vi "水温校准.vi"() -> ()   [LabVIEW 2016, in "斯坦道多参数.lvlib"]
uses:
  <vilib>/Utility/miscctls.llb/LVPointTypeDef.ctl
  <vilib>/Utility/miscctls.llb/LVPositionTypeDef.ctl
  <vilib>/Utility/miscctls.llb/LVBoundsTypeDef.ctl
  <vilib>/Utility/config.llb/NI_LVConfig.lvlib
panel:
  out "字符串":string
  in  "补偿后温度值":dbl format="%#_g ℃"
  out "电极温度读值":dbl format="%#_g ℃"
  in  "温度偏移补偿":dbl format="%#_g ℃"
  in  "温度电极选择":enum16{"pH电极", "电导率电极", "溶解氧电极", "浊度电极"}(ring)
  # "温度电极设定"
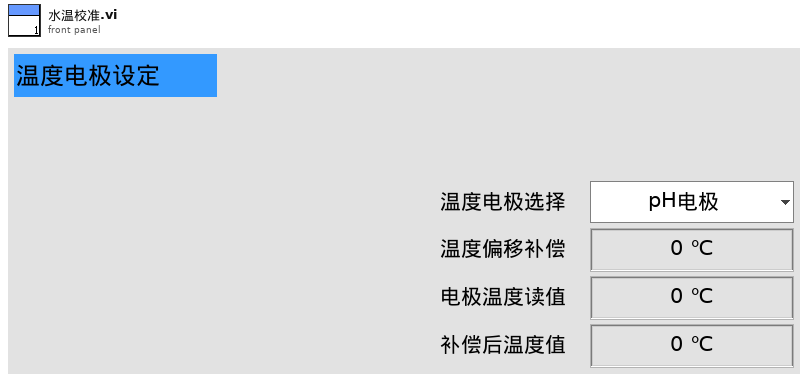
[diagram p1: front panel]
types:
  T1 = typedef "LVPointTypeDef.ctl" = cluster{"Horizontal":i16, "Vertical":i16}
  T2 = typedef "LVPositionTypeDef.ctl" = cluster{"Left":i32, "Top":i32}
  T3 = typedef "LVBoundsTypeDef.ctl" = cluster{"Width":u32, "Height":u32}
  T4 = cluster{"pH探头选择":u16, "DO探头选择":u16, "电导率探头选择":u16, "浊度探头选择":u16, "叶绿素a探头选择":u16, "蓝绿藻探头选择":u16, "orp探头选择":u16}
  T5 = cluster{"CH":u16, "监测值":dbl, "温度偏移修正值":sgl, "信号值":sgl}
  T6 = typedef "NI_LVConfig.lvlib/Config Data RefNum.ctl" = refnum<k1>
  T7 = cluster{"报警码":u16, "pH数值":sgl, "0X0003_NC":sgl, "温度数据":sgl, "pH原始信号 mv":sgl, "0X0009_NC":string, "产品名称":string, "序列号":string, "硬件版本":string, "软件版本":string, "通讯地址":u16, "波特率":u16, "设备类型":u16, "0X0026_NC":string, "第一点原始数据":sgl, "第一点校准数据":sgl, "第二点原始数据":sgl, "第二点校准数据":sgl, "探头校准命令":u16, "温度校准参数":sgl, "温度校准命令":u16}
  T8 = cluster{"报警码":u16, "电导率数据（uS/cm）":sgl, "0x0003 NC":sgl, "温度数据":sgl, "电导率原始信号电阻":sgl, "当前量程":u16, "温度补偿系数":sgl, "0X0009_NC":string, "产品名称":string, "序列号":string, "硬件版本":string, "软件版本":string, "通讯地址":u16, "波特率":u16, "设备类型":u16, "0X0026_NC":string, "第一点原始数据":sgl, "第一点校准数据":sgl, "0X0035_NC":sgl, "0X0037_NC":sgl, "探头校准命令":u16, "温度校准参数":sgl, "温度校准命令":u16}
  T9 = cluster{"报警码":u16, "溶解氧数值（mg/L）":sgl, "溶解氧数据（%）":sgl, "温度数据":sgl, "溶解氧原始信号 nA":sgl, "大气压力":sgl, "盐度":sgl, "0X0009_NC":string, "产品名称":string, "序列号":string, "硬件版本":string, "软件版本":string, "通讯地址":u16, "波特率":u16, "设备类型":u16, "0X0026_NC":string, "第一点原始数据":sgl, "第一点校准数据":sgl, "第二点原始数据":sgl, "第二点校准数据":sgl, "探头校准命令":u16, "温度校准参数":sgl, "温度校准命令":u16}
  T10 = cluster{"报警码":u16, "浊度数值 NTU":sgl, "温度数据":sgl, "原始光强数值":u16, "量程":u16, "平均次数":u16, "清扫模式":u16, "清扫次数":u16, "清扫间隔分钟":u16, "0X000B_NC":string, "产品名称":string, "序列号":string, "硬件版本":string, "软件版本":string, "通讯地址":u16, "波特率":u16, "设备类型":u16, "0X0026_NC":string, "校准量程":u16, "第一点原始光强":u16, "第一点校准数据":sgl, "第二点原始光强":u16, "第二点校准数据":sgl, "第三点原始光强":u16, "第三点校准数据":sgl, "探头校准命令":u16, "温度校准参数":sgl, "温度校准命令":u16}
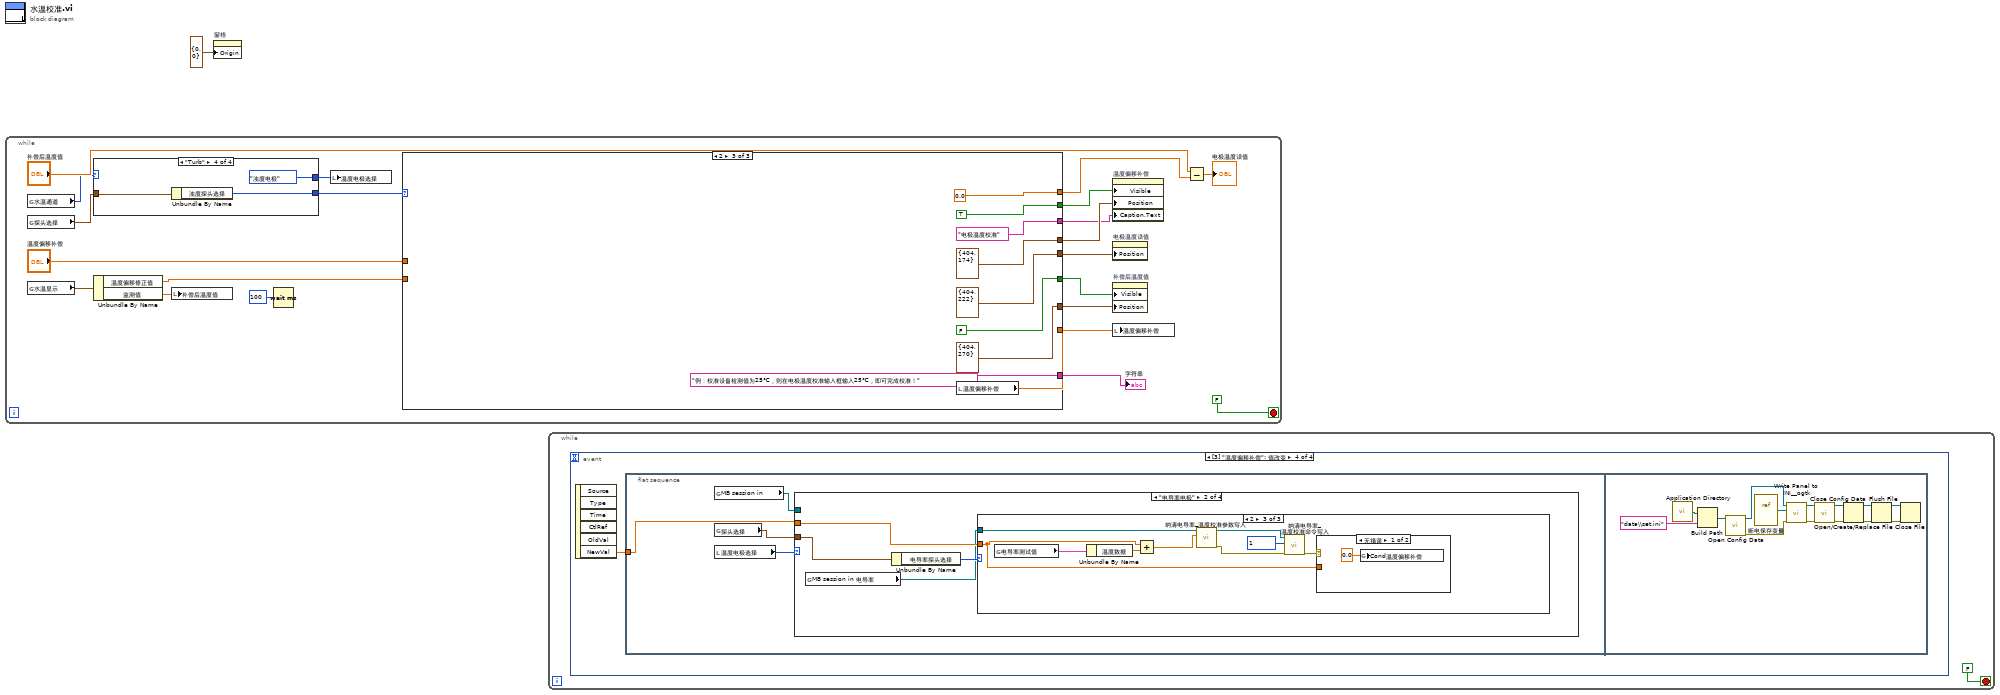
[diagram p0: block diagram]
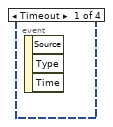
[diagram p2: hidden frame]
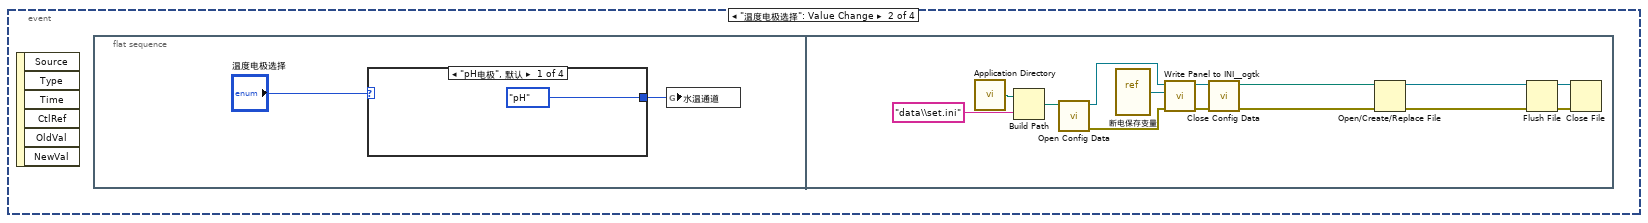
[diagram p3: hidden frame]
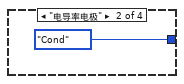
[diagram p4: hidden frame]
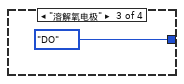
[diagram p5: hidden frame]
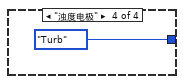
[diagram p6: hidden frame]
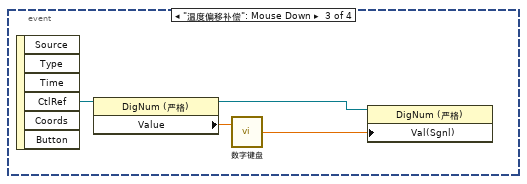
[diagram p7: hidden frame]
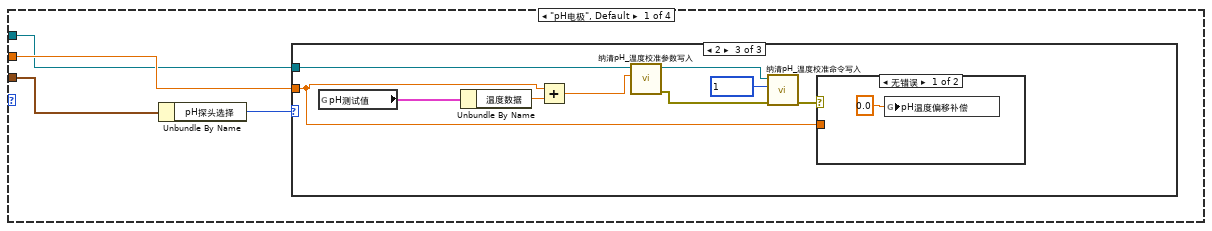
[diagram p8: hidden frame]
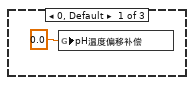
[diagram p9: hidden frame]
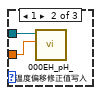
[diagram p10: hidden frame]
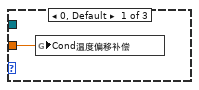
[diagram p12: hidden frame]
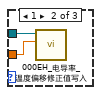
[diagram p13: hidden frame]
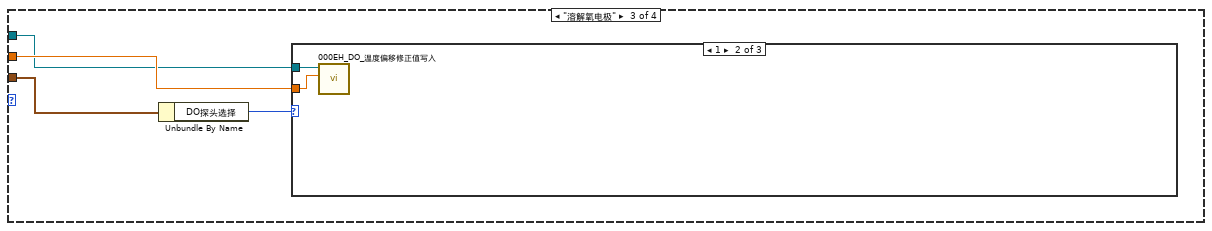
[diagram p15: hidden frame]
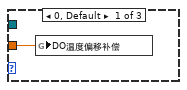
[diagram p16: hidden frame]
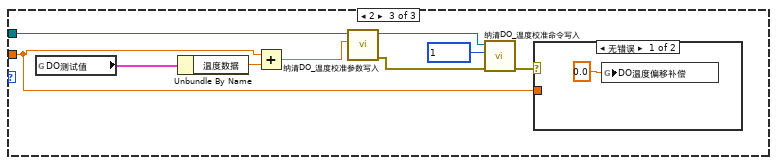
[diagram p17: hidden frame]
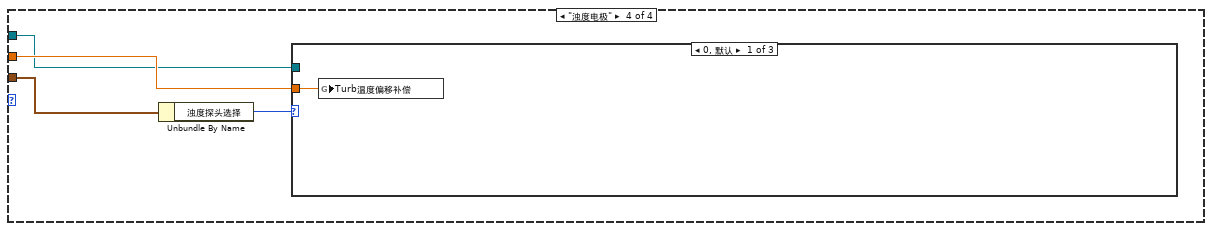
[diagram p19: hidden frame]
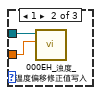
[diagram p20: hidden frame]
diagram:
  n1 = while {
    stop <- FALSE stop-if-true
    n2 = global read "断电保存变量.vi" "水温通道"() -> (w17:enum16{"pH", "Cond", "DO", "Turb"})
    n3 = global read "断电保存变量.vi" "探头选择"() -> (w14:T4)
    n4 = global read "多参数全局变量.vi" "水温显示"() -> (w16:T5)
    n5 = case shown="\"Turb\"" w17 {
      tunnel: [enum16{"pH电极", "电导率电极", "溶解氧电极", "浊度电极"}."pH电极" ("温度电极选择") enum16{"pH电极", "电导率电极", "溶解氧电极", "浊度电极"}."电导率电极" ("温度电极选择") enum16{"pH电极", "电导率电极", "溶解氧电极", "浊度电极"}."溶解氧电极" ("温度电极选择") enum16{"pH电极", "电导率电极", "溶解氧电极", "浊度电极"}."浊度电极" ("温度电极选择")] -> w15
      tunnel: w14 -> [w50 w53 w56 w59]
      tunnel: [w49 w52 w55 w58] -> w13
      frame "pH", Default {
        n6 = Unbundle By Name(w50) -> ("pH探头选择"=w49:u16)
      }
      frame "Cond" {
        n7 = Unbundle By Name(w53) -> ("电导率探头选择"=w52:u16)
      }
      frame "DO" {
        n8 = Unbundle By Name(w56) -> ("DO探头选择"=w55:u16)
      }
      frame "Turb" {
        n9 = Unbundle By Name(w59) -> ("浊度探头选择"=w58:u16)
      }
    }
    n10 = Unbundle By Name(w16) -> ("温度偏移修正值"=w6:sgl, "监测值"=w18:dbl)
    n11 = local write "补偿后温度值"(w18) -> ()
    n12 = Wait (ms)(milliseconds to wait=u32 100 ("等待时间（毫秒）")) -> ()  [unwired: 1 out]
    n13 = local write "温度电极选择"(w15) -> ()
    n14 = case shown="2" w13 {
      tunnel: [FALSE ("可见") TRUE ("可见") TRUE ("可见")] -> w12
      tunnel: [w29 T2 {"Left"=404, "Top"=174} ("位置") T2 {"Left"=404, "Top"=174} ("位置")] -> w11
      tunnel: [w29 T3 {"Width"=404, "Height"=222} ("边界") T3 {"Width"=404, "Height"=222} ("边界")] -> w10
      tunnel: [FALSE ("可见") TRUE ("可见") FALSE ("可见")] -> w9
      tunnel: [T2 {"Left"=404, "Top"=270} ("位置 2") T2 {"Left"=404, "Top"=270} ("位置 2") T2 {"Left"=404, "Top"=270} ("位置 2")] -> w8
      tunnel: ["温度偏移补偿" ("标题.文本") "温度偏移补偿" ("标题.文本") "电极温度校准" ("标题.文本")] -> w7
      tunnel: w6 -> [w25 w33 _]
      tunnel: [w25 w33 w42] -> w5
      tunnel: "温度偏移补偿" -> [w24 w32 _]
      tunnel: [w24 w32 0.0 ("温度偏移补偿")] -> w3
      tunnel: ["此探头温度不可校准！" ("字符串") "例：校准设备检测值为25℃，电极温度读值为24.5℃，则在温度偏移补偿输入框输入0.5℃（25-24.5），即可完成校准！" ("字符串") "例：校准设备检测值为25℃，则在电极温度校准输入框输入25℃，即可完成校准！" ("字符串")] -> w2
      frame 0, Default {
        (unwired) T3 {"Width"=404, "Height"=222} ("边界")
        w29 = T2 {"Left"=404, "Top"=174} ("位置")
      }
      frame 1 {
      }
      frame 2 {
        n15 = local read "温度偏移补偿"() -> (w42:dbl)
      }
    }
    "字符串" <- w2
    n16 = property on="温度偏移补偿" class="DigNum (严格)"("Visible"=w12, "Position"=w11, "Caption.Text"=w7) -> ()  [unwired: 2 in, 2 out]
    n17 = property on="电极温度读值" class="DigNum (严格)"("Position"=w10) -> ()  [unwired: 2 in, 2 out]
    n18 = property on="补偿后温度值" class="DigNum (严格)"("Visible"=w9, "Position"=w8) -> ()  [unwired: 2 in, 2 out]
    n19 = local write "温度偏移补偿"(w5) -> ()
    n20 = Subtract(x="补偿后温度值", y=w3) -> (x-y=→"电极温度读值":dbl)
  }
  n21 = property on="窗格" class="Pane"("Origin"=T1 {"Horizontal"=0, "Vertical"=0} ("原点")) -> ()  [unwired: 2 in, 2 out]
  n22 = while {
    stop <- FALSE stop-if-true
    n23 = event shown="[3] \"温度偏移补偿\": 值改变" {
      selector: _ -> [_ _ _ _]
      dyn-events: _ -> [_ _ _ _]
      timeout: _ -> [_ _ _ _]
      event Timeout {
        n24 = event-data() -> ()  [unwired: 1 in, 3 out]
      }
      event "温度电极选择": Value Change {
        n25 = event-data() -> ()  [unwired: 1 in, 6 out]
        n26 = flat-sequence {
          frame #0 {
            n27 = case shown="\"pH电极\", 默认" "温度电极选择" {
              tunnel: [enum16{"pH", "Cond", "DO", "Turb"}."pH" ("水温通道") enum16{"pH", "Cond", "DO", "Turb"}."Cond" ("水温通道") enum16{"pH", "Cond", "DO", "Turb"}."DO" ("水温通道") enum16{"pH", "Cond", "DO", "Turb"}."Turb" ("水温通道")] -> w63
              frame "pH电极", Default {
              }
              frame "电导率电极" {
              }
              frame "溶解氧电极" {
              }
              frame "浊度电极" {
              }
            }
            n28 = global write "断电保存变量.vi" "水温通道"(w63) -> ()
          }
          frame #1 {
            n29 = call <vilib>:"Application Directory.vi"() -> ("Application Directory"=w77:path)
            n30 = Build Path(base path=w77, name or relative path="data\\set.ini" ("名称或相对路径")) -> (appended path=w76:path)
            n31 = call <vilib>:"Open Config Data.vi"("configuration file path"=w76) -> ("error out"=w80:errorcluster, "refnum"=w81:T6)  [unwired: 8 in, 1 out]
            n32 = vi-ref "断电保存变量.vi"() -> (w74:refnum<vi>)
            n33 = call <userlib>:"Write Panel to INI__ogtk.vi"("error in (no error)"=w80, "VI ref"=w74, "refnum"=w81) -> ("error out"=w78:errorcluster, "refnum out"=w79:T6)  [unwired: 7 in]
            n34 = call <vilib>:"Close Config Data.vi"("error in (no error)"=w78, "refnum"=w79) -> ("error out"=w70:errorcluster, "file path"=w71:path)  [unwired: 8 in]
            n35 = Open/Create/Replace File(file path (use dialog)=w71, error in=w70) -> (refnum out=w72:refnum<file>, error out=w73:errorcluster)  [unwired: 4 in, 1 out]
            n36 = Flush File(refnum=w72, error in=w73) -> (refnum out=w68:refnum<file>, error out=w69:errorcluster)
            n37 = Close File(refnum=w68, error in=w69) -> ()  [unwired: 2 out]
          }
        }
      }
      event "温度偏移补偿": Mouse Down {
        n38 = event-data() -> ("CtlRef"=w85:refnum<vi>)  [unwired: 1 in, 5 out]
        n39 = property class="DigNum (严格)"(reference=w85) -> (reference out=w82:refnum<vi>, "Value"=w84:dbl)  [unwired: 1 in, 1 out]
        n40 = call "数字键盘.vi"("OldNumber"=w84) -> ("NewNumber"=w83:dbl)  [unwired: 1 in]
        n41 = property class="DigNum (严格)"(reference=w82, "Val(Sgnl)"=w83) -> ()  [unwired: 1 in, 2 out]
      }
      event "温度偏移补偿": Value Change {
        n42 = event-data() -> ("NewVal"=w86:dbl)  [unwired: 1 in, 5 out]
        n43 = flat-sequence {
          tunnel: w86 -> [w89]
          frame #0 {
            n44 = global read "多参数全局变量.vi" "MB session in"() -> (w88:refnum<class "MB_Master.lvclass">)
            n45 = global read "断电保存变量.vi" "探头选择"() -> (w87:T4)
            n46 = local read "温度电极选择"() -> (w90:enum16{"pH电极", "电导率电极", "溶解氧电极", "浊度电极"})
            n47 = case shown="\"电导率电极\"" w90 {
              tunnel: w89 -> [w94 w111 w128 w145]
              tunnel: w88 -> [w93 _ w125 w142]
              tunnel: w87 -> [w92 w110 w127 w144]
              frame "pH电极", Default {
                n48 = Unbundle By Name(w92) -> ("pH探头选择"=w91:u16)
                n49 = case shown="2" w91 {
                  tunnel: w94 -> [_ w97 w98]
                  tunnel: w93 -> [_ w96 w100]
                  frame 0, Default {
                    n50 = global write "断电保存变量.vi" "pH温度偏移补偿"(0.0 ("pH温度偏移补偿")) -> ()
                  }
                  frame 1 {
                    n51 = call "000EH_pH_温度偏移修正值写入.vi"("数值"=w97, "MB session in"=w96) -> ()  [unwired: 8 in, 2 out]
                  }
                  frame 2 {
                    n52 = global read "纳清过程全局变量.vi" "pH测试值"() -> (w106:T7)
                    n53 = Unbundle By Name(w106) -> ("温度数据"=w105:sgl)
                    n54 = Add(x=w98, y=w105) -> (x+y=w101:dbl)
                    n55 = call "纳清pH_温度校准参数写入.vi"("数值"=w101, "MB session in"=w100) -> ("error out"=w102:errorcluster, "MB session out"=w103:refnum<class "MB_Master.lvclass">)  [unwired: 8 in]
                    n56 = call "纳清pH_温度校准命令写入.vi"("error in (no error)"=w102, "数值"=u16 1 ("starting address"), "MB session in"=w103) -> ("error out"=w99:errorcluster)  [unwired: 7 in, 1 out]
                    n57 = case shown="无错误" w99 {
                      tunnel: w98 -> [_ _]
                      frame No Error {
                        n58 = global write "断电保存变量.vi" "pH温度偏移补偿"(0.0 ("pH温度偏移补偿")) -> ()
                      }
                      frame Error {
                      }
                    }
                  }
                }
              }
              frame "电导率电极" {
                n59 = global read "多参数全局变量.vi" "MB session in 电导率"() -> (w108:refnum<class "MB_Master.lvclass">)
                n60 = Unbundle By Name(w110) -> ("电导率探头选择"=w109:u16)
                n61 = case shown="2" w109 {
                  tunnel: w111 -> [w112 w114 w115]
                  tunnel: w108 -> [_ w113 w120]
                  frame 0, Default {
                    n62 = global write "断电保存变量.vi" "Cond温度偏移补偿"(w112) -> ()
                  }
                  frame 1 {
                    n63 = call "000EH_电导率_温度偏移修正值写入.vi"("数值"=w114, "MB session in"=w113) -> ()  [unwired: 8 in, 2 out]
                  }
                  frame 2 {
                    n64 = global read "纳清过程全局变量.vi" "电导率测试值"() -> (w119:T8)
                    n65 = Unbundle By Name(w119) -> ("温度数据"=w118:sgl)
                    n66 = Add(x=w115, y=w118) -> (x+y=w117:dbl)
                    n67 = call "纳清电导率_温度校准参数写入.vi"("数值"=w117, "MB session in"=w120) -> ("error out"=w123:errorcluster, "MB session out"=w122:refnum<class "MB_Master.lvclass">)  [unwired: 8 in]
                    n68 = call "纳清电导率_温度校准命令写入.vi"("error in (no error)"=w123, "数值"=u16 1 ("starting address"), "MB session in"=w122) -> ("error out"=w116:errorcluster)  [unwired: 7 in, 1 out]
                    n69 = case shown="无错误" w116 {
                      tunnel: w115 -> [_ _]
                      frame No Error {
                        n70 = global write "断电保存变量.vi" "Cond温度偏移补偿"(0.0 ("Cond温度偏移补偿")) -> ()
                      }
                      frame Error {
                      }
                    }
                  }
                }
              }
              frame "溶解氧电极" {
                n71 = Unbundle By Name(w127) -> ("DO探头选择"=w126:u16)
                n72 = case shown="1" w126 {
                  tunnel: w128 -> [w129 w130 w132]
                  tunnel: w125 -> [_ w131 w137]
                  frame 0, Default {
                    n73 = global write "断电保存变量.vi" "DO温度偏移补偿"(w129) -> ()
                  }
                  frame 1 {
                    n74 = call "000EH_DO_温度偏移修正值写入.vi"("数值"=w130, "MB session in"=w131) -> ()  [unwired: 8 in, 2 out]
                  }
                  frame 2 {
                    n75 = global read "纳清过程全局变量.vi" "DO测试值"() -> (w136:T9)
                    n76 = Unbundle By Name(w136) -> ("温度数据"=w135:sgl)
                    n77 = Add(x=w132, y=w135) -> (x+y=w134:dbl)
                    n78 = call "纳清DO_温度校准参数写入.vi"("数值"=w134, "MB session in"=w137) -> ("error out"=w140:errorcluster, "MB session out"=w139:refnum<class "MB_Master.lvclass">)  [unwired: 8 in]
                    n79 = call "纳清DO_温度校准命令写入.vi"("error in (no error)"=w140, "数值"=u16 1 ("starting address"), "MB session in"=w139) -> ("error out"=w133:errorcluster)  [unwired: 7 in, 1 out]
                    n80 = case shown="无错误" w133 {
                      tunnel: w132 -> [_ _]
                      frame No Error {
                        n81 = global write "断电保存变量.vi" "DO温度偏移补偿"(0.0 ("DO温度偏移补偿")) -> ()
                      }
                      frame Error {
                      }
                    }
                  }
                }
              }
              frame "浊度电极" {
                n82 = Unbundle By Name(w144) -> ("浊度探头选择"=w143:u16)
                n83 = case shown="0, 默认" w143 {
                  tunnel: w145 -> [w146 w148 w149]
                  tunnel: w142 -> [_ w147 w153]
                  frame 0, Default {
                    n84 = global write "断电保存变量.vi" "Turb温度偏移补偿"(w146) -> ()
                  }
                  frame 1 {
                    n85 = call "000EH_浊度_温度偏移修正值写入.vi"("数值"=w148, "MB session in"=w147) -> ()  [unwired: 8 in, 2 out]
                  }
                  frame 2 {
                    n86 = global read "纳清过程全局变量.vi" "浊度测试值"() -> (w157:T10)
                    n87 = Unbundle By Name(w157) -> ("温度数据"=w152:sgl)
                    n88 = Add(x=w149, y=w152) -> (x+y=w151:dbl)
                    n89 = call "纳清叶绿素a_温度校准参数写入.vi"("数值"=w151, "MB session in"=w153) -> ("error out"=w154:errorcluster, "MB session out"=w155:refnum<class "MB_Master.lvclass">)  [unwired: 8 in]
                    n90 = call "纳清叶绿素a_温度校准命令写入.vi"("error in (no error)"=w154, "数值"=u16 1 ("starting address"), "MB session in"=w155) -> ("error out"=w150:errorcluster)  [unwired: 7 in, 1 out]
                    n91 = case shown="无错误" w150 {
                      tunnel: w149 -> [_ _]
                      frame No Error {
                        n92 = global write "断电保存变量.vi" "Turb温度偏移补偿"(0.0 ("Turb温度偏移补偿")) -> ()
                      }
                      frame Error {
                      }
                    }
                  }
                }
              }
            }
          }
          frame #1 {
            n93 = call <vilib>:"Application Directory.vi"() -> ("Application Directory"=w168:path)
            n94 = Build Path(base path=w168, name or relative path="data\\set.ini" ("名称或相对路径")) -> (appended path=w167:path)
            n95 = call <vilib>:"Open Config Data.vi"("configuration file path"=w167) -> ("error out"=w171:errorcluster, "refnum"=w172:T6)  [unwired: 8 in, 1 out]
            n96 = vi-ref "断电保存变量.vi"() -> (w165:refnum<vi>)
            n97 = call <userlib>:"Write Panel to INI__ogtk.vi"("error in (no error)"=w171, "VI ref"=w165, "refnum"=w172) -> ("error out"=w169:errorcluster, "refnum out"=w170:T6)  [unwired: 7 in]
            n98 = call <vilib>:"Close Config Data.vi"("error in (no error)"=w169, "refnum"=w170) -> ("error out"=w161:errorcluster, "file path"=w162:path)  [unwired: 8 in]
            n99 = Open/Create/Replace File(file path (use dialog)=w162, error in=w161) -> (refnum out=w163:refnum<file>, error out=w164:errorcluster)  [unwired: 4 in, 1 out]
            n100 = Flush File(refnum=w163, error in=w164) -> (refnum out=w159:refnum<file>, error out=w160:errorcluster)
            n101 = Close File(refnum=w159, error in=w160) -> ()  [unwired: 2 out]
          }
        }
      }
    }
  }
